vi "CaptStub.vi"(6 "Graph in":cluster{dbl[], dbl[]}, 8 "error in":errorcluster, 9 "Length":i32=250, 11 "ON":bool) -> (0 "error out":errorcluster, 2 "Values":cluster{dbl[], dbl[]})   [LabVIEW 2013]
uses:
  GlobalVariables/CalibrationState.vi
  GlobalVariables/CalibrationVolumes.vi
  GlobalVariables/PressureAndTimeSamples.vi
  GlobalVariables/ValveValues.vi
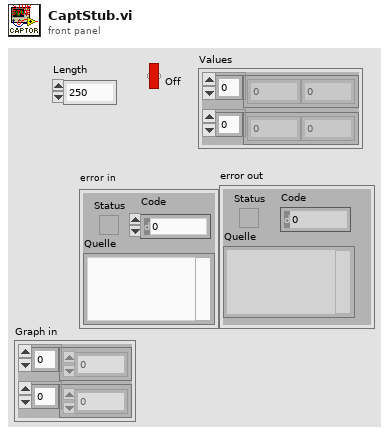
[diagram p1: front panel]
types:
  T1 = cluster{"TimeSamples":dbl[], "PressureSamples":dbl[]}
  T2 = cluster{bool, "CalibrationStep":u32, "Volumes":dbl[], "PressureRatios":dbl[]}
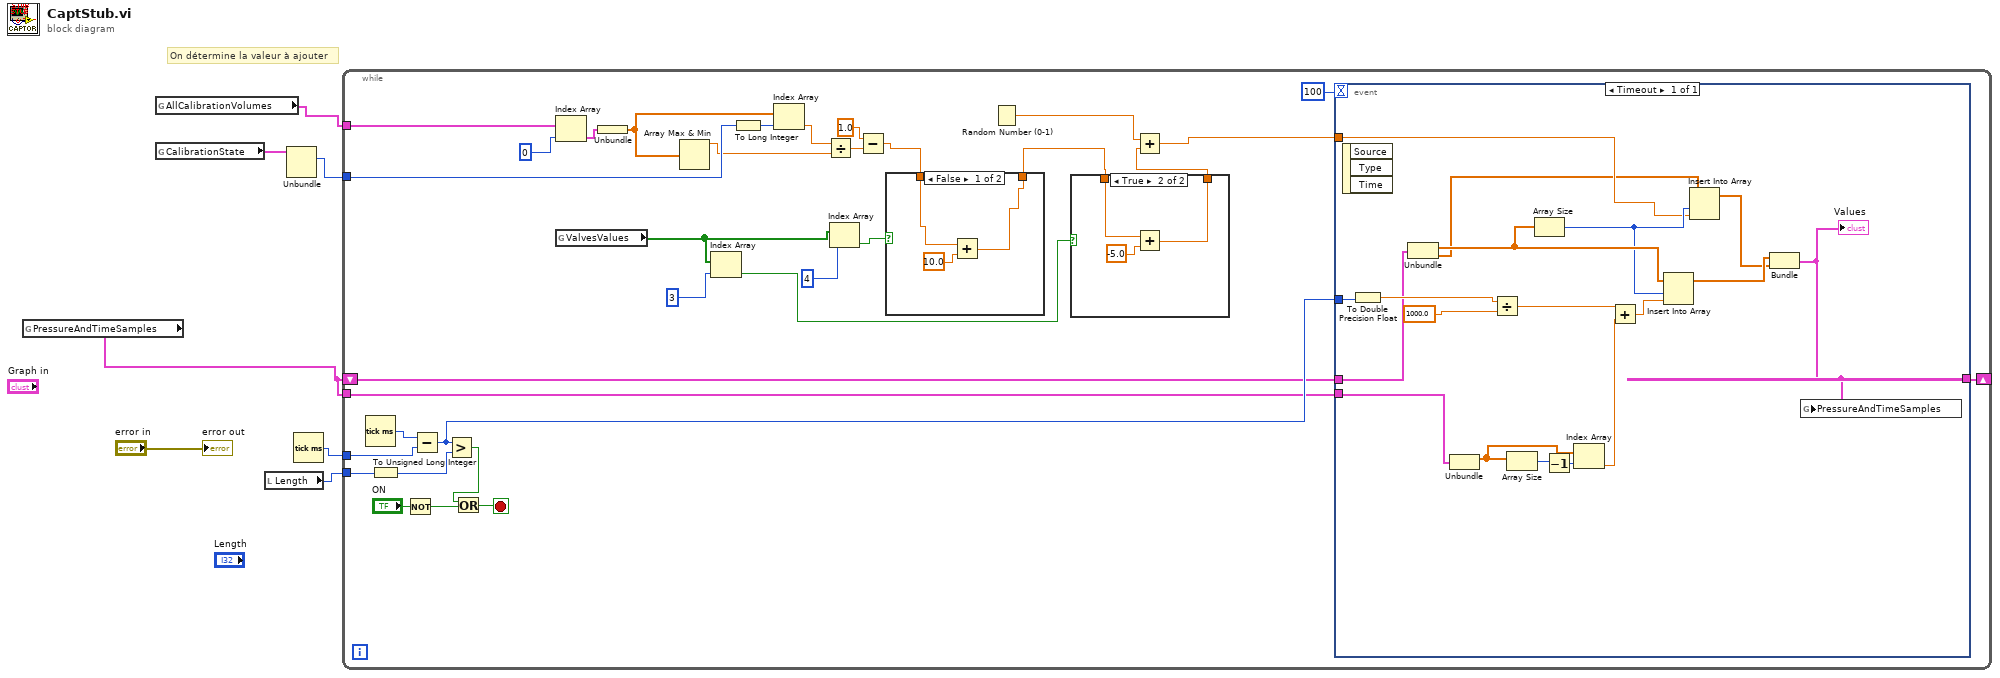
[diagram p0: block diagram]
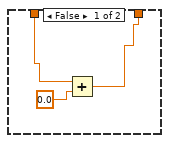
[diagram p2: hidden frame]
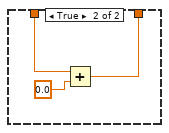
[diagram p3: hidden frame]
diagram:
  # "On détermine la valeur à ajouter"
  n1 = global read "PressureAndTimeSamples.vi" "PressureAndTimeSamples"() -> (w1:T1)
  n2 = global read "CalibrationVolumes.vi" "AllCalibrationVolumes"() -> (w3:cluster{"CalibrationVolumes":dbl[]}[])
  n3 = global read "CalibrationState.vi" "CalibrationState"() -> (w4:T2)
  n4 = local read "Length"() -> (w6:i32)
  n5 = Unbundle(w4) -> ("CalibrationStep"=w2:u32)  [unwired: 3 out]
  n6 = Tick Count (ms)() -> (millisecond timer value=w7:u32)
  n7 = while {
    tunnel: w7 -> [w36]
    tunnel: w6 -> [w31]
    shift-right: [w29] -> _
    shift-left: w1 -> [w32]
    tunnel: w3 -> [w27]
    tunnel: w2 -> [w26]
    tunnel: w1 -> [w8]
    stop <- w38 stop-if-true
    n8 = Tick Count (ms)() -> (millisecond timer value=w37:u32)
    n9 = To Unsigned Long Integer(number=w31) -> (unsigned 32bit integer=w30:u32)
    n10 = Not(x="ON") -> (.not. x?=w39:bool)
    n11 = Subtract(x=w37, y=w36) -> (x-y=w33:u32)
    n12 = Greater?(x=w33, y=w30) -> (0:w35:bool)
    n13 = Or(x=w35, y=w39) -> (x .or. y?=w38:bool)
    n14 = Index Array(array=w27, index=0) -> (element=w19:cluster{"CalibrationVolumes":dbl[]})
    n15 = global read "ValveValues.vi" "ValvesValues"() -> (w13:bool[])
    n16 = Unbundle(w19) -> ("CalibrationVolumes"=w18:dbl[])
    n17 = Array Max & Min(array=w18) -> (max value=w21:dbl)  [unwired: 3 out]
    n18 = Index Array(array=w13, index=3) -> (element=w11:bool)
    n19 = To Long Integer(number=w26) -> (32bit integer=w25:i32)
    n20 = Index Array(array=w18, index=w25) -> (element=w22:dbl)
    n21 = Divide(x=w22, y=w21) -> (x/y=w23:dbl)
    n22 = Index Array(array=w13, index=4) -> (element=w16:bool)
    n23 = Subtract(x=1.0, y=w23) -> (x-y=w14:dbl)
    n24 = case shown="False" w16 {
      tunnel: w14 -> [w48 w52]
      tunnel: [w47 w51] -> w10
      frame False {
        n25 = Add(x=w48, y=10.0) -> (x+y=w47:dbl)
      }
      frame True {
        n26 = Add(x=w52, y=0.0) -> (x+y=w51:dbl)
      }
    }
    n27 = Random Number (0-1)() -> (number: 0 to 1=w17:dbl)
    n28 = case shown="True" w11 {
      tunnel: w10 -> [w42 w46]
      tunnel: [w41 w45] -> w9
      frame False {
        n29 = Add(x=w42, y=0.0) -> (x+y=w41:dbl)
      }
      frame True {
        n30 = Add(x=w46, y=-5.0) -> (x+y=w45:dbl)
      }
    }
    n31 = Add(x=w17, y=w9) -> (x+y=w28:dbl)
    n32 = event shown="[0] Timeout" {
      selector: _ -> [_]
      dyn-events: _ -> [_]
      timeout: 100 -> [_]
      tunnel: w33 -> [w60]
      tunnel: w32 -> [w54]
      tunnel: [w55] -> w29
      tunnel: w28 -> [w58]
      tunnel: w8 -> [w53]
      event Timeout {
        n33 = event-data() -> ()  [unwired: 1 in, 3 out]
        n34 = To Double Precision Float(number=w60) -> (double precision float=w59:dbl)
        n35 = Unbundle(w54) -> ("TimeSamples"=w62:dbl[], "PressureSamples"=w57:dbl[])
        n36 = Unbundle(w53) -> ("TimeSamples"=w68:dbl[])  [unwired: 1 out]
        n37 = Divide(x=w59, y=1000.0) -> (x/y=w64:dbl)
        n38 = Array Size(array=w68) -> (size(s)=w70:i32)
        n39 = Array Size(array=w62) -> (size(s)=w61:i32)
        n40 = Decrement(x=w70) -> (x-1=w69:i32)
        n41 = Index Array(array=w68, index=w69) -> (element=w56:dbl)
        n42 = Add(x=w64, y=w56) -> (x+y=w63:dbl)
        n43 = Insert Into Array(array=w62, index=w61, new element=w63) -> (w66:dbl[])
        n44 = Insert Into Array(array=w57, index=w61, new element=w58) -> (w65:dbl[])
        n45 = Bundle("TimeSamples"=w66, "PressureSamples"=w65) -> (w55:T1)  [unwired: 1 in]
        "Values" <- w55
        n46 = global write "PressureAndTimeSamples.vi" "PressureAndTimeSamples"(w55) -> ()
      }
    }
  }
  "error out" <- "error in"
